vi "datatakersync_master.vi"() -> ()   [LabVIEW 2014, in "filenames.lvlib"]
doc: "This example demonstrates how to acquire a single buffer of voltage measurements using a DAQmx device.\n\nFor instructions on how to connect your signals to the DAQ device, refer to your device documentation."
uses:
  filenames.lvlib
  <resource>/objmgr/daqmx.rc
  <vilib>/DAQmx/configure/timing.llb/DAQmx Timing (Sample Clock).vi
  <vilib>/Utility/error.llb/DialogType.ctl
  <vilib>/DAQmx/create/channels.llb/DAQmx Create Channel (AI-Voltage-Basic).vi
  <vilib>/DAQmx/configure/trigger.llb/DAQmx Start Trigger (Digital Edge).vi
  <vilib>/ptbypt/NI_PtbyPt.lvlib
  <userlib>/Agilis Labview 7.1/AGILIS.llb/enter / leave remote mode.vi
  <vilib>/DAQmx/create/channels.llb/DAQmx Create Channel (AO-Voltage-Basic).vi
  <vilib>/DAQmx/write.llb/DAQmx Write (Analog 1D DBL 1Chan NSamp).vi
  <vilib>/LabVIEW Hacker/LINX/Public/Peripherals/Analog/Analog Read 1 Chan.vi
  <vilib>/Analysis/3filter.llb/Filter Passband Type.ctl
  <vilib>/Analysis/NI_AALBase.lvlib
panel:
  in  "Agilent is negative?":bool
  in  "Set Agilent DC":bool
  in  "stop (DC)":ext=1.0
  in  "start (DC)":ext=1.0
  in  "Number of DC steps":i32=1
  in  "Jog during auto":bool=TRUE
  in  "Move Slide Back 3":bool
  in  "Move Slide  2":bool
  in  "Slide Jog Speed 2":i32(slide) scale=1.0..3.0
  in  "Stop Button":bool=TRUE
  in  "Use interferometer":bool
  out "Motion Direction Indicator":bool
  out "Move Indicator":bool
  in  "Auto Move":bool=TRUE
  in  "Auto Motion Direction":bool
  in  "Tab Control":T1(tab)=enum."I/O"
  out "Indicator Pos 2":bool
  out "Indicator Pos 1":bool=TRUE
  in  "Go to 2":bool
  in  "Go to 1":bool
  in  "Cycles Between Movements":i32=1
  in  "Position 2":dbl=2.5
  in  "Position 1":dbl=-2.5
  out "Main Sig":dbl[][](graph)=[[-1.679588746006175], [-2.01550649520741]]
  out "Main Output":dbl(graph)=1.3000000000000012
  out "Displacement":dbl=1.3000000000000012 format="%#.3f"
  in  "Zero":bool
  in  "Go to Zero":bool
  in  "Automatic":bool
  in  "Motion Direction":bool=TRUE
  in  "Manual Move":bool
  in  "Stop Movement":bool
  in  "Arduino Serial Port":refnum<visa-resource-name>="COM3"
  out "Device Name":string="Arduino Mega 2560"
  in  "Analog Channel":u8
  out "Filtered Signal":dbl(graph)=-1.679588746006175
  in  "filter type":T2=enum."Bandpass"
  in  "order":i32=2
  in  "initialize":bool
  in  "low cutoff freq: fl":dbl=0.45 format="%#_13g"
  out "Raw Signal":dbl(graph)=2.294921875
  in  "Positive Move Steps":i32=30
  in  "Controller Serial Port":u8=6
  in  "Negative Move Steps":i32=30
  in  "Move Period (ms)":u32=10
  in  "high cutoff freq: fh":dbl=1.0
  out "Input Signals":dbl[][](graph)=[[-1.679588746006175], [-2.01550649520741]]
  out "Stepped Signal":dbl(graph)=2.0
  in  "Fringe Counter Settings":T3={"Wavelength"=3.25e-07, "Divisions"=2.0, "Scaling Amplitude"=1.2, "Scaling Offset"=0.0} {"Scaling Offset" format="%0.2f"; "Scaling Amplitude" format="%0.2f"}
  out "Fringe Counter Output Signal":dbl[](graph)=[1.21875e-06]
  out "Relative Displacement":dbl=1.21875e-06
  out "Total Displacement":dbl(graph)=1.3000000000000012
  out "Reset Fringe Counter":bool
  out "Timeout":bool
  in  "Slide Jog Speed":i32(slide) scale=1.0..3.0
  in  "Move Slide":bool
  in  "Move Slide Back":bool
  in  "Error In":errorcluster
  in  "Turn off drive\nwhen flashing?":bool
  in  "set synth":bool
  in  "Sweep type":u16(ring)=1 items=["Chirp", "Single freq", "Both"]
  in  "VISA session":refnum<visa-resource-name>="GPIB0::10::INSTR"
  in  "Physical Channel synth_trigger":tag="Dev5/ao0"
  in  "Digitize on\nother comp?":bool
  in  "stop (F)":ext=100.0
  in  "start (F)":ext=100.0
  in  "Number of F Steps":i32=1
  in  "dc offset?":bool
  in  "volt_div":dbl=200.0
  in  "stop (V)":ext=0.05
  in  "start (V)":ext=0.05
  in  "Number of V Steps":i32=1
  out "error out":errorcluster
  in  "Physical Channel (drive signals)":tag="Dev5/ai0"
  out "Curr threshold":dbl
  in  "Stop threshold":dbl=0.05
  in  "Stop flashing below thresh":bool
  out "Pirani pressure (mbar)":string
  out "CC read error":errorcluster={"status"=FALSE, "code"=1073676294, "source"="VISA Read in read_pressure(SubVI).vi->hdf5(SubVI).vi->filenames.lvlib:datatakersync_master.vi"}
  out "CC pressure (mbar)":string
  out "Pirani read error":errorcluster={"status"=FALSE, "code"=1073676294, "source"="VISA Read in read_pressure(SubVI).vi->hdf5(SubVI).vi->filenames.lvlib:datatakersync_master.vi"}
  in  "# Pulses":i32=3
  in  "Output channel (for flashing)":tag="Dev4/ao0"
  in  "Number of cyles\nbetween flashes":i32=3
  in  "Flash lamp?":bool
  in  "File base name":string="2mbar_zcool"
  in  "Delay time between files(s)":dbl caption="Delay Time (s)"
  in  "Num files":i32=1
  out "Temps (C):":dbl[](array[numeric])
  in  "VISA Refnum in":refnum<visa-resource-name>="GPIB0::19::INSTR"
  in  "Directory path":path=path "D:/Data/20150528/Bead1"
  out "Waveform Graph":dbl[][](graph)
  in  "Number of Samples":i32=100000
  in  "Sample Rate":dbl=10000.0
  in  "Sample Clock Source":tag="/Dev2/PXI_Clk10"
  in  "Terminal Configuration":i32(ring)=-1 items=["default"=-1, "RSE"=10083, "NRSE"=10078, "Differential"=10106, "Pseudodifferential"=12529]
  in  "Max Voltage":dbl=10.0
  in  "Physical Channels (Position signals)":tag="Dev2/ai0:7"
  out "Actual Sample Rate":dbl=10000.0 format="%0.2f"
  # "Channel Settings"
  # "Acquired Data"
  # "Timing Settings"
  # "Flash Lamp Settings"
  # "Pressures and Temperatures"
  # "Logging Settings"
  # "."
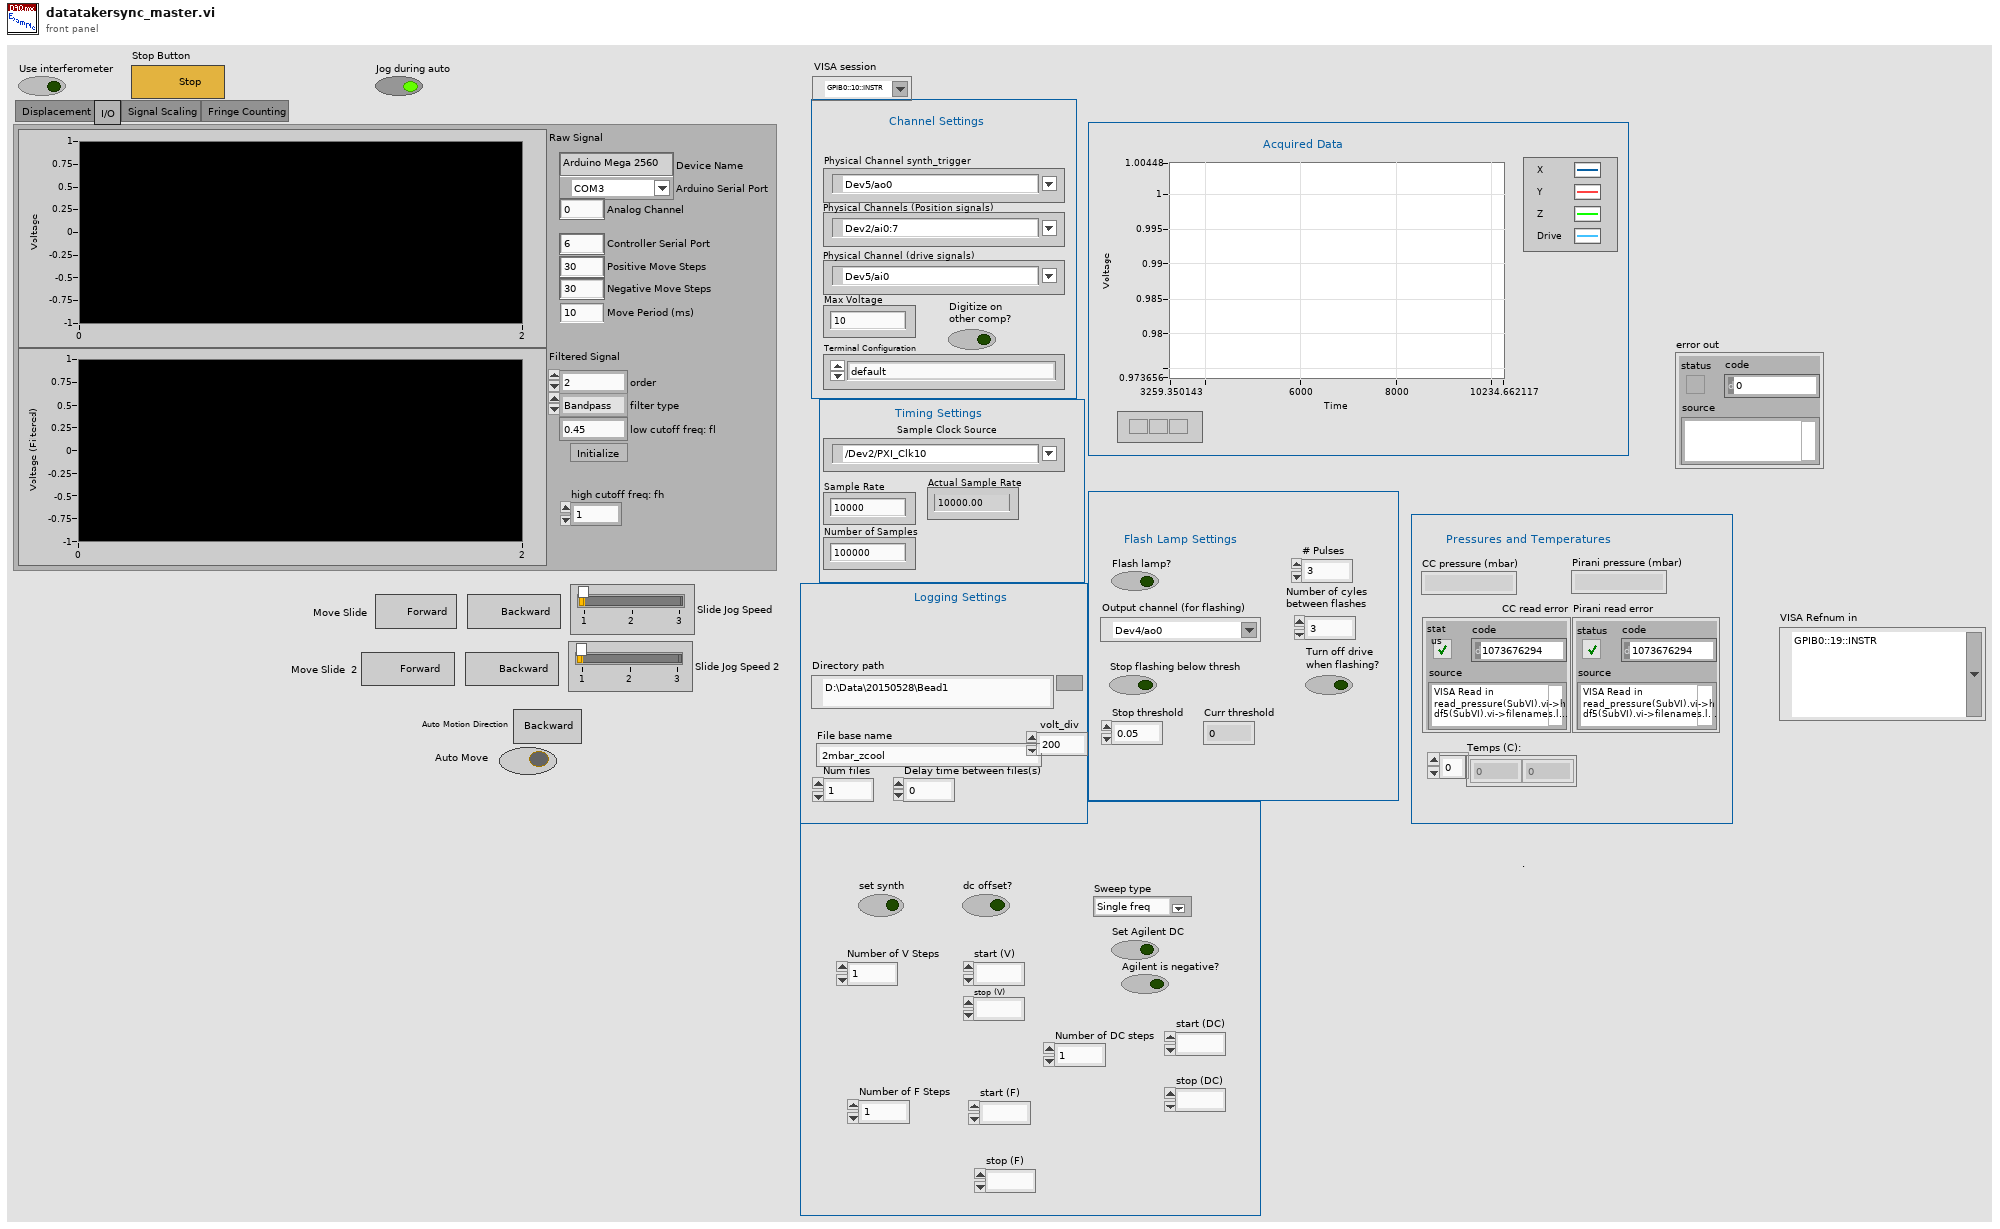
[diagram p1: front panel]
types:
  T1 = enum32{"Displacement", "I/O", "Signal Scaling", "Fringe Counting"}
  T2 = typedef "NI_AALBase.lvlib/Filter Passband Type.ctl" = enum32{"Lowpass", "Highpass", "Bandpass", "Bandstop"}
  T3 = cluster{"Wavelength":dbl, "Divisions":dbl, "Scaling Amplitude":dbl, "Scaling Offset":dbl}
  T4 = typedef "DialogType.ctl" = u16
  T5 = typedef "LVH-LINX.lvlib/LINX Ref.ctl" = cluster{"Platform":T6, "Interface":T7, "LINX Device Config":T8}
  T6 = typedef "LVH-LINX.lvlib/Platform.ctl" = enum16{"LINX", "myRIO"}
  T7 = typedef "LVH-LINX.lvlib/Interface.ctl" = enum16{"Serial", "TCP"}
  T8 = typedef "LVH-LINX.lvlib/Device.lvlib/LINX Device Config.ctl" = cluster{"Interface":T7, "COM Port":refnum<visa-resource-name>, "TCP Configuration":T9, "Device Family":T10, "Device ID":u8, "Device Name":string, "TCP Ref":refnum<k5>}
  T9 = typedef "LVH-LINX.lvlib/Device.lvlib/TCP Config.ctl" = cluster{"IP Address":string, "Port":u16}
  T10 = typedef "LVH-LINX.lvlib/Device Family.ctl" = enum8{"National Instruments", "Digilent", "Arduino"}
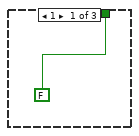
[diagram p3: hidden frame]
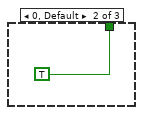
[diagram p4: hidden frame]
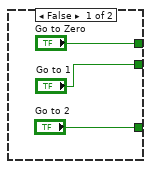
[diagram p5: hidden frame]
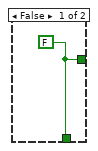
[diagram p6: hidden frame]
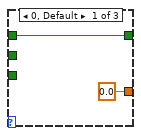
[diagram p8: hidden frame]
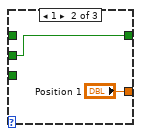
[diagram p9: hidden frame]
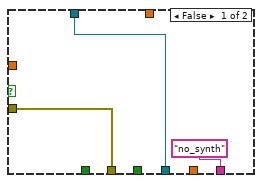
[diagram p11: hidden frame]
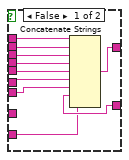
[diagram p12: hidden frame]
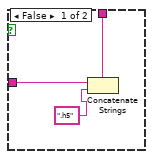
[diagram p14: hidden frame]
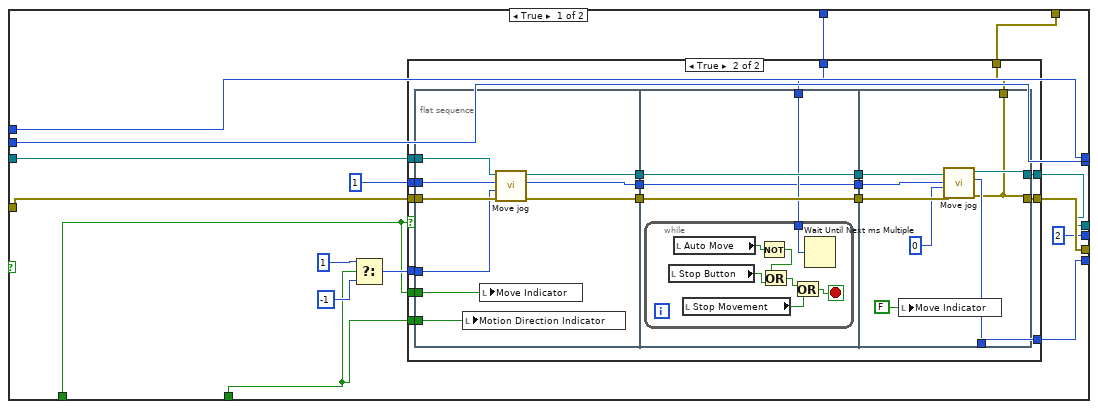
[diagram p18: hidden frame]
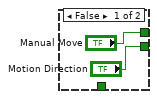
[diagram p20: hidden frame]
diagram:
  w17 = TRUE  # ID Query
  w52 = 10178 items=["Finite Samples"=10178, "Continuous Samples"=10123, "Hardware Timed Single Point"=12522]  # Sample Mode
  n1 = case shown="True" "set synth" {
    tunnel: w17 -> [_ w60]
    tunnel: [refnum<visa-resource-name> refnum ("dup VISA session") w57] -> w16
    tunnel: [errorcluster {"status"=FALSE, "code"=0, "source"=""} ("error out") w56] -> w15
    frame False {
    }
    frame True {
      n2 = call "ag33xxx - Initialize.vi"("ID Query (T: Check)"=w60, "Instrument Resource Name"="VISA session") -> ("error out"=w59:errorcluster, "dup VISA session"=w58:refnum<visa-resource-name>)  [unwired: 8 in]
      n3 = VISA Write(VISA resource name=w58, write buffer="SOUR:BM:NCYC INF;:SOUR:BM:PHAS 0;SOUR INT;:TRIG:SOUR EXT;:SOUR:BM:INT:RATE 1.000000;:BM:STAT ON;", error in (no error)=w59) -> (VISA resource name out=w57:refnum<visa-resource-name>, error out=w56:errorcluster)  [unwired: 1 out]
    }
  }
  n4 = call <vilib>:"Check if File or Folder Exists.vi"("path"="Directory path") -> ("file or folder exists?"=w42:bool, "dup path"=w41:path)  [unwired: 8 in, 1 out]
  n5 = Subtract(x="stop (DC)", y="start (DC)") -> (x-y=w5:ext)
  n6 = case shown="False" w42 {
    tunnel: w41 -> [w63 w68]
    tunnel: [w62 w68] -> w40
    frame False {
      n7 = flat-sequence {
        tunnel: w63 -> [w67]
        tunnel: [w66] -> w62
        frame #0 {
          n8 = call "Create folder?"() -> ("OK"=w65:bool)  [unwired: 18 in, 1 out]
          n9 = Not(x=w65) -> (.not. x?=w64:bool)
          n10 = Stop(stop? (T)=w64) -> ()
        }
        frame #1 {
          n11 = Create Folder(path (use dialog)=w67) -> (created path=w66:path)  [unwired: 2 in, 2 out]
        }
      }
    }
    frame True {
    }
  }
  n12 = Subtract(x="stop (F)", y="start (F)") -> (x-y=w28:ext)
  n13 = Divide(x=w5, y="Number of DC steps") -> (x/y=w4:ext)
  n14 = Divide(x=w28, y="Number of F Steps") -> (x/y=w27:ext)
  n15 = Subtract(x="stop (V)", y="start (V)") -> (x-y=w35:ext)
  n16 = Multiply(x="Max Voltage", y=-1.0) -> (x*y=w45:dbl)
  n17 = Divide(x=w35, y="Number of V Steps") -> (x/y=w33:ext)
  n18 = case shown="True" "Digitize on\nother comp?" {
    selector: "Digitize on\nother comp?" -> [w69 w72]
    tunnel: [errorcluster {"status"=FALSE, "code"=0, "source"=""} ("error out") w75] -> w24
    tunnel: [refnum<k5> refnum ("connection ID") w74] -> w23
    tunnel: [w69 w72] -> w19
    frame False {
    }
    frame True {
      w76 = 60000  # timeout ms
      n19 = call <vilib>:"TCP Listen.vi"("timeout ms (wait forever: -1)"=w76, "port"=u16 6340) -> ("error out"=w75:errorcluster, "connection ID"=w74:refnum<k5>)  [unwired: 5 in, 3 out]
    }
  }
  n20 = local write "Automatic"(FALSE ("Go to Zero")) -> ()
  n21 = for {
    N: "Number of DC steps" -> [_]
    tunnel: w52 -> [w116]
    tunnel: "Physical Channels (Position signals)" -> [w115]
    tunnel: "Terminal Configuration" -> [w114]
    tunnel: "Sample Clock Source" -> [w113]
    tunnel: "Sample Rate" -> [w112]
    tunnel: "Number of Samples" -> [w111]
    tunnel: w45 -> [w110]
    tunnel: "Max Voltage" -> [w109]
    tunnel: w40 -> [w108]
    tunnel: "File base name" -> [w107]
    tunnel: "Output channel (for flashing)" -> [w106]
    tunnel: "Physical Channel (drive signals)" -> [w105]
    tunnel: "Number of V Steps" -> [w104]
    tunnel: w33 -> [w103]
    tunnel: "start (V)" -> [w102]
    tunnel: "Num files" -> [w101]
    tunnel: "volt_div" -> [w100]
    tunnel: w27 -> [w99]
    tunnel: "start (F)" -> [w98]
    tunnel: "Number of F Steps" -> [w97]
    tunnel: w24 -> [w96]
    tunnel: w23 -> [w95]
    tunnel: [w94] -> w22
    tunnel: [w93] -> w21
    tunnel: w19 -> [w92]
    tunnel: [w91] -> w7
    tunnel: "Physical Channel synth_trigger" -> [w90]
    tunnel: w16 -> [w89]
    tunnel: w15 -> [w88]
    tunnel: [w87] -> w14
    tunnel: [w86] -> w13
    tunnel: [w85] -> w12
    tunnel: "Sweep type" -> [w84]
    tunnel: "set synth" -> [w83]
    tunnel: "start (DC)" -> [w81]
    tunnel: w4 -> [w79]
    tunnel: [w77] -> w1
    i -> [w82]
    n22 = Multiply(x=w79, y=w82) -> (x*y=w80:ext)
    n23 = Add(x=w81, y=w80) -> (x+y=w78:ext)
    n24 = for {
      N: w101 -> [_]
      tunnel: w116 -> [w156]
      tunnel: w115 -> [w155]
      tunnel: w114 -> [w154]
      tunnel: w113 -> [w153]
      tunnel: w112 -> [w152]
      tunnel: w111 -> [w151]
      tunnel: w110 -> [w150]
      tunnel: w109 -> [w149]
      tunnel: w108 -> [w148]
      tunnel: w107 -> [w147]
      tunnel: w106 -> [w146]
      tunnel: w105 -> [w145]
      tunnel: w104 -> [w144]
      tunnel: w103 -> [w143]
      tunnel: w102 -> [w142]
      tunnel: w101 -> [w141]
      tunnel: w83 -> [w140]
      tunnel: w100 -> [w139]
      tunnel: w99 -> [w138]
      tunnel: w98 -> [w137]
      tunnel: w97 -> [w136]
      tunnel: w96 -> [w135]
      tunnel: w95 -> [w134]
      tunnel: [w133] -> w94
      tunnel: [w132] -> w93
      tunnel: w92 -> [w131]
      tunnel: [w130] -> w91
      tunnel: w90 -> [w129]
      tunnel: w89 -> [w128]
      tunnel: w88 -> [w127]
      tunnel: [w126] -> w87
      tunnel: [w125] -> w86
      tunnel: [w124] -> w85
      tunnel: w83 -> [w123]
      tunnel: w84 -> [w121]
      tunnel: w78 -> [w119]
      tunnel: [w117] -> w77
      i -> [w120]
      n25 = case shown="2" w121 {
        tunnel: [FALSE TRUE w159] -> w122
        tunnel: w120 -> [_ _ w163]
        frame 1 {
        }
        frame 0, Default {
        }
        frame 2 {
          n26 = Quotient & Remainder(x=w163, y=2) -> (x-y*floor(x/y)=w161:i32)  [unwired: 1 out]
          n27 = Equal?(x=w161, y=0) -> (x = y?=w159:bool)
        }
      }
      n28 = for {
        N: w144 -> [_]
        tunnel: w156 -> [w203]
        tunnel: w155 -> [w202]
        tunnel: w154 -> [w201]
        tunnel: w153 -> [w200]
        tunnel: w152 -> [w199]
        tunnel: w151 -> [w198]
        tunnel: w150 -> [w197]
        tunnel: w149 -> [w196]
        tunnel: w148 -> [w195]
        tunnel: w147 -> [w194]
        tunnel: w146 -> [w193]
        tunnel: w145 -> [w192]
        tunnel: w143 -> [w191]
        tunnel: w142 -> [w190]
        tunnel: w120 -> [w188]
        tunnel: w141 -> [w187]
        tunnel: w140 -> [w186]
        tunnel: w139 -> [w185]
        tunnel: w138 -> [w184]
        tunnel: w137 -> [w183]
        tunnel: w136 -> [w182]
        tunnel: w122 -> [w181]
        tunnel: w135 -> [w180]
        tunnel: w134 -> [w179]
        tunnel: [w178] -> w133
        tunnel: [w177] -> w132
        tunnel: w131 -> [w176]
        tunnel: [w175] -> w130
        tunnel: w129 -> [w174]
        tunnel: w128 -> [w173]
        tunnel: w127 -> [w172]
        tunnel: [w171] -> w126
        tunnel: [w170] -> w125
        tunnel: [w169] -> w124
        tunnel: w123 -> [w168]
        tunnel: w120 -> [w167]
        tunnel: w119 -> [w166]
        tunnel: "Set Agilent DC" -> [w165]
        tunnel: [w164] -> w117
        i -> [w189]
        n29 = for {
          N: w182 -> [_]
          tunnel: w203 -> [w344]
          tunnel: w202 -> [w343]
          tunnel: w201 -> [w342]
          tunnel: w200 -> [w341]
          tunnel: w199 -> [w269]
          tunnel: w198 -> [w340]
          tunnel: w197 -> [w339]
          tunnel: w196 -> [w338]
          tunnel: w195 -> [w337]
          tunnel: w194 -> [w336]
          tunnel: w193 -> [w335]
          tunnel: w192 -> [w334]
          tunnel: w191 -> [w333]
          tunnel: w190 -> [w331]
          tunnel: w189 -> [w329]
          tunnel: w188 -> [w328]
          tunnel: w187 -> [w297]
          tunnel: w186 -> [w327]
          tunnel: w185 -> [w326]
          tunnel: w184 -> [w322]
          tunnel: w183 -> [w321]
          tunnel: w181 -> [w319]
          tunnel: w180 -> [w318]
          tunnel: w179 -> [w317]
          tunnel: [w316] -> w178
          tunnel: [w315] -> w177
          tunnel: w176 -> [w314]
          tunnel: [w313] -> w175
          tunnel: w174 -> [w268]
          tunnel: w173 -> [w264]
          tunnel: w172 -> [w263]
          tunnel: [w259] -> w171
          tunnel: [w255] -> w170
          tunnel: [w254] -> w169
          tunnel: w168 -> [w250]
          tunnel: w167 -> [w212]
          tunnel: w166 -> [w211]
          tunnel: w165 -> [w208]
          tunnel: [w204] -> w164
          i -> [w320]
          n30 = Multiply(x=w322, y=w320) -> (x*y=w323:ext)
          n31 = Add(x=w321, y=w323) -> (x+y=w324:ext)
          n32 = Multiply(x=w329, y=w333) -> (x*y=w332:ext)
          n33 = Add(x=w331, y=w332) -> (x+y=w330:ext)
          n34 = flat-sequence {
            tunnel: w250 -> [w353]
            tunnel: w263 -> [w354]
            tunnel: w264 -> [w355]
            tunnel: w268 -> [w356]
            tunnel: w314 -> [w357]
            tunnel: w317 -> [w358]
            tunnel: w318 -> [w359]
            tunnel: w319 -> [w360]
            tunnel: "dc offset?" -> [w361]
            tunnel: w327 -> [w362]
            tunnel: w328 -> [w363]
            tunnel: w330 -> [w364]
            tunnel: w330 -> [w365]
            tunnel: w324 -> [w366]
            tunnel: w334 -> [w367]
            tunnel: w335 -> [w368]
            tunnel: w336 -> [w369]
            tunnel: w337 -> [w370]
            tunnel: w338 -> [w371]
            tunnel: w339 -> [w372]
            tunnel: w341 -> [w373]
            tunnel: w342 -> [w374]
            tunnel: w343 -> [w375]
            tunnel: [w375] -> w235
            tunnel: [w374] -> w234
            tunnel: [w373] -> w233
            tunnel: [w372] -> w232
            tunnel: [w371] -> w231
            tunnel: [w370] -> w230
            tunnel: [w369] -> w229
            tunnel: [w368] -> w228
            tunnel: [w367] -> w227
            tunnel: [w366] -> w226
            tunnel: [w365] -> w225
            tunnel: [w364] -> w224
            tunnel: [w363] -> w223
            tunnel: [w362] -> w222
            tunnel: [w361] -> w221
            tunnel: [w360] -> w220
            tunnel: [w359] -> w219
            tunnel: [w358] -> w218
            tunnel: [w357] -> w217
            tunnel: [w356] -> w216
            tunnel: [w355] -> w215
            tunnel: [w354] -> w214
            tunnel: [w353] -> w213
            tunnel: w212 -> [w346]
            tunnel: w211 -> [w345]
            tunnel: [w345] -> w210
            tunnel: [w454] -> w301
            tunnel: [w453] -> w302
            tunnel: [w452] -> w303
            tunnel: [w451] -> w304
            tunnel: [w450] -> w305
            tunnel: [w449] -> w306
            tunnel: [w448] -> w307
            tunnel: [w447] -> w308
            tunnel: [w446] -> w309
            tunnel: [w444] -> w310
            tunnel: [w443] -> w311
            tunnel: [w442] -> w312
            tunnel: [w440] -> w300
            tunnel: [w439] -> w299
            tunnel: [w438] -> w298
            tunnel: [w437] -> w267
            tunnel: [w434] -> w262
            tunnel: [w433] -> w258
            tunnel: [w432] -> w251
            tunnel: [w431] -> w246
            tunnel: [w430] -> w245
            tunnel: [w429] -> w240
            tunnel: w235 -> [w454]
            tunnel: w234 -> [w453]
            tunnel: w233 -> [w452]
            tunnel: w232 -> [w451]
            tunnel: w231 -> [w450]
            tunnel: w230 -> [w449]
            tunnel: w229 -> [w448]
            tunnel: w228 -> [w447]
            tunnel: w227 -> [w446]
            tunnel: w226 -> [w444]
            tunnel: w225 -> [w445]
            tunnel: w224 -> [w443]
            tunnel: w223 -> [w442]
            tunnel: w222 -> [w441]
            tunnel: w221 -> [w429]
            tunnel: w220 -> [w431]
            tunnel: w219 -> [w440]
            tunnel: w218 -> [w439]
            tunnel: w217 -> [w438]
            tunnel: w216 -> [w437]
            tunnel: w215 -> [w436]
            tunnel: w214 -> [w435]
            tunnel: w213 -> [w432]
            tunnel: w210 -> [w428]
            tunnel: [w428] -> w209
            tunnel: w208 -> [w427]
            tunnel: [w427] -> w207
            tunnel: w312 -> [w523]
            tunnel: w311 -> [w493]
            tunnel: w310 -> [w528]
            tunnel: [w528] -> w296
            tunnel: w309 -> [w537]
            tunnel: [w537] -> w294
            tunnel: w308 -> [w536]
            tunnel: [w536] -> w292
            tunnel: w307 -> [w502]
            tunnel: w306 -> [w504]
            tunnel: w305 -> [w535]
            tunnel: [w535] -> w289
            tunnel: w304 -> [w534]
            tunnel: [w534] -> w287
            tunnel: w303 -> [w533]
            tunnel: [w533] -> w285
            tunnel: w302 -> [w532]
            tunnel: [w532] -> w283
            tunnel: w301 -> [w531]
            tunnel: [w531] -> w281
            tunnel: w300 -> [w513]
            tunnel: [w510] -> w279
            tunnel: w299 -> [w514]
            tunnel: [w511] -> w277
            tunnel: w298 -> [w512]
            tunnel: [w509] -> w275
            tunnel: [w529] -> w273
            tunnel: w297 -> [w526]
            tunnel: [w523] -> w271
            tunnel: w267 -> [w508]
            tunnel: [w508] -> w265
            tunnel: w262 -> [w507]
            tunnel: [w507] -> w260
            tunnel: w258 -> [w506]
            tunnel: [w506] -> w256
            tunnel: [w505] -> w253
            tunnel: w251 -> [w505]
            tunnel: [w504] -> w249
            tunnel: [w503] -> w248
            tunnel: w246 -> [w496]
            tunnel: w245 -> [w495]
            tunnel: [w496] -> w243
            tunnel: [w495] -> w242
            tunnel: w240 -> [w494]
            tunnel: [w494] -> w239
            tunnel: [w493] -> w237
            tunnel: w209 -> [w491]
            tunnel: w207 -> [w487]
            tunnel: [w487] -> w205
            tunnel: w296 -> [w602]
            tunnel: [w602] -> w295
            tunnel: w294 -> [w601]
            tunnel: [w601] -> w293
            tunnel: w292 -> [w600]
            tunnel: [w600] -> w291
            tunnel: [w599] -> w290
            tunnel: w289 -> [w598]
            tunnel: [w598] -> w288
            tunnel: w287 -> [w597]
            tunnel: [w597] -> w286
            tunnel: w285 -> [w596]
            tunnel: [w596] -> w284
            tunnel: w283 -> [w595]
            tunnel: [w595] -> w282
            tunnel: w281 -> [w589]
            tunnel: [w589] -> w280
            tunnel: w279 -> [w594]
            tunnel: [w594] -> w278
            tunnel: w277 -> [w593]
            tunnel: [w593] -> w276
            tunnel: w275 -> [w592]
            tunnel: [w592] -> w274
            tunnel: w273 -> [w591]
            tunnel: [w591] -> w272
            tunnel: w271 -> [w590]
            tunnel: [w590] -> w270
            tunnel: [w588] -> w266
            tunnel: w265 -> [w588]
            tunnel: [w587] -> w261
            tunnel: w260 -> [w587]
            tunnel: [w586] -> w257
            tunnel: w256 -> [w586]
            tunnel: w253 -> [w585]
            tunnel: [w585] -> w252
            tunnel: w249 -> [w599]
            tunnel: w248 -> [w584]
            tunnel: [w584] -> w247
            tunnel: [w583] -> w244
            tunnel: w243 -> [w583]
            tunnel: w242 -> [w582]
            tunnel: [w582] -> w241
            tunnel: w239 -> [w581]
            tunnel: [w581] -> w238
            tunnel: w237 -> [w580]
            tunnel: [w580] -> w236
            tunnel: [w579] -> w206
            tunnel: w205 -> [w579]
            tunnel: w344 -> [w706]
            tunnel: w269 -> [w626]
            tunnel: w340 -> [w703]
            tunnel: w326 -> [w656]
            tunnel: w295 -> [w616]
            tunnel: w293 -> [w699]
            tunnel: w291 -> [w700]
            tunnel: w290 -> [w650]
            tunnel: w288 -> [w701]
            tunnel: w286 -> [w702]
            tunnel: w284 -> [w648]
            tunnel: w282 -> [w704]
            tunnel: w280 -> [w705]
            tunnel: w278 -> [w652]
            tunnel: w276 -> [w653]
            tunnel: [w652] -> w316
            tunnel: [w653] -> w315
            tunnel: w274 -> [w651]
            tunnel: [w651] -> w313
            tunnel: w272 -> [w655]
            tunnel: w270 -> [w654]
            tunnel: w266 -> [w649]
            tunnel: w261 -> [w611]
            tunnel: [w610] -> w259
            tunnel: w257 -> [w615]
            tunnel: [w609] -> w255
            tunnel: [w634] -> w254
            tunnel: w252 -> [w634]
            tunnel: w247 -> [w633]
            tunnel: w244 -> [w614]
            tunnel: w241 -> [w613]
            tunnel: w238 -> [w612]
            tunnel: w236 -> [w608]
            tunnel: w206 -> [w603]
            tunnel: [w603] -> w204
            frame #0 {
              n35 = case shown="True" "Automatic" {
                tunnel: w346 -> [_ w386]
                tunnel: ["Go to Zero" FALSE ("Go to Zero")] -> w349
                tunnel: ["Go to 1" w380] -> w350
                tunnel: ["Go to 2" w381] -> w351
                frame False {
                }
                frame True {
                  n36 = Quotient & Remainder(x=w386, y="Cycles Between Movements") -> (x-y*floor(x/y)=w384:i32, floor(x/y)=w382:i32)
                  n37 = Equal To 0?(x=w384) -> (x = 0?=w383:bool)
                  n38 = case shown="True" w383 {
                    tunnel: w382 -> [_ w392]
                    tunnel: [w387 w389] -> w381
                    tunnel: [w387 w388] -> w380
                    frame False {
                      w387 = FALSE
                    }
                    frame True {
                      n39 = Quotient & Remainder(x=w392, y=2) -> (x-y*floor(x/y)=w390:i32)  [unwired: 1 out]
                      n40 = Equal To 0?(x=w390) -> (x = 0?=w388:bool)
                      n41 = Not(x=w388) -> (.not. x?=w389:bool)
                    }
                  }
                }
              }
              n42 = local read "Displacement"() -> (w348:dbl)
              n43 = for {
                N: 3 -> [_]
                tunnel: w349 -> [w398]
                tunnel: w350 -> [w395]
                tunnel: w351 -> [w394]
                tunnel: w348 -> [w396]
                i -> [w399]
                n44 = case shown="2" w399 {
                  tunnel: w398 -> [w422 _ _]
                  tunnel: w395 -> [_ w424 _]
                  tunnel: w394 -> [_ _ w426]
                  tunnel: [w422 w424 w426] -> w393
                  tunnel: [0.0 ("Position 2") "Position 1" "Position 2"] -> w397
                  frame 0, Default {
                  }
                  frame 1 {
                  }
                  frame 2 {
                  }
                }
                n45 = case shown="True" w393 {
                  tunnel: w397 -> [_ w406]
                  tunnel: w396 -> [_ w405]
                  tunnel: w395 -> [_ w401]
                  tunnel: w394 -> [_ w402]
                  tunnel: w393 -> [_ w400]
                  frame False {
                  }
                  frame True {
                    n46 = Greater?(x=w406, y=w405) -> (0:w404:bool)
                    n47 = local write "Auto Motion Direction"(w404) -> ()
                    n48 = local write "Auto Move"(w400) -> ()
                    n49 = while {
                      tunnel: w406 -> [w407]
                      tunnel: w404 -> [w419]
                      tunnel: w402 -> [w416]
                      tunnel: w401 -> [w415]
                      tunnel: [FALSE] -> w403
                      stop <- w412 stop-if-true
                      n50 = local read "Displacement"() -> (w408:dbl)
                      n51 = Not Equal?(x=w408, y=w407) -> (x != y?=w409:bool)
                      n52 = Greater?(x=w407, y=w408) -> (0:w420:bool)
                      n53 = Equal?(x=w420, y=w419) -> (x = y?=w414:bool)
                      n54 = And(x=w409, y=w414) -> (x .and. y?=w410:bool)
                      n55 = And(x=w415, y=w410) -> (x .and. y?=→"Indicator Pos 1":bool)
                      n56 = And(x=w416, y=w410) -> (x .and. y?=→"Indicator Pos 2":bool)
                      n57 = Compound Arithmetic op=OR(invert w410, "Stop Movement") -> (w412:bool)
                    }
                    n58 = local write "Auto Move"(w403) -> ()
                  }
                }
              }
            }
            frame #1 {
              n59 = case shown="True" w441 {
                tunnel: w445 -> [_ w471]
                tunnel: w444 -> [_ w470]
                tunnel: w429 -> [_ w469]
                tunnel: w431 -> [_ w468]
                tunnel: w436 -> [w460 w467]
                tunnel: w435 -> [w461 w466]
                tunnel: [w461 w465] -> w434
                tunnel: [w460 w464] -> w433
                tunnel: ["no_synth" ("User Def. Wfm Name") w463] -> w430
                tunnel: w428 -> [_ w462]
                frame False {
                }
                frame True {
                  n60 = flat-sequence {
                    tunnel: w471 -> [w481]
                    tunnel: w470 -> [w480]
                    tunnel: w469 -> [w479]
                    tunnel: w468 -> [w478]
                    tunnel: w467 -> [w477]
                    tunnel: w466 -> [w473]
                    tunnel: [w472] -> w465
                    tunnel: [w476] -> w464
                    tunnel: [w475] -> w463
                    tunnel: w462 -> [w474]
                    frame #0 {
                      w475 = "RANDFREQ" ("User Def. Wfm Name")
                      n61 = call "synth_set(SubVI).vi"("dc offset?"=w479, "dc offset"=w474, "error in (no error)"=w473, "User Def. Wfm Name"=w475, "chirp?"=w478, "VISA session"=w477, "amplitude (V)"=w481, "frequency (Hz)"=w480) -> ("dup VISA session"=w476:refnum<visa-resource-name>, "error out"=w472:errorcluster)  [unwired: 2 in]
                    }
                    frame #1 {
                      n62 = call "Time Delay2"() -> ()  [unwired: 11 in, 1 out]
                    }
                  }
                }
              }
              n63 = case shown="True" w427 {
                tunnel: w428 -> [_ w458]
                frame False {
                }
                frame True {
                  n64 = call <instrlib>:"Agilent E364X Series Output Single Channel DC Volts.vi"("VISA resource name"=refnum<visa-resource-name> "GPIB0::8::INSTR", "Output Enabled (False)"=TRUE, "Voltage Level (0.0 Volts)"=w458, "Current Limit (0 Amps)"=0.01) -> ()  [unwired: 11 in, 1 out]
                }
              }
            }
            frame #2 {
              n65 = Multiply(x=w493, y=ext 1000.0) -> (x*y=w529:ext)
              n66 = Multiply(x=w491, y=ext 1000.0) -> (x*y=w490:ext)
              n67 = Number To Decimal String(number=w490) -> (decimal integer string=w484:string)  [unwired: 1 in]
              n68 = Number To Decimal String(number=w529) -> (decimal integer string=w500:string)  [unwired: 1 in]
              n69 = Number To Decimal String(number=w528) -> (decimal integer string=w498:string)  [unwired: 1 in]
              n70 = Concatenate Strings("-" ("string"), w484) -> (w483:string)
              n71 = Select(t=w483, s="Agilent is negative?", f=w484) -> (s? t:f=w486:string)
              n72 = case shown="True" w496 {
                tunnel: [w547 w551] -> w524
                tunnel: w502 -> [w546 w556]
                tunnel: "_" ("string") -> [w545 w555]
                tunnel: w500 -> [w544 w554]
                tunnel: "mV_" ("string") -> [w543 w553]
                tunnel: w498 -> [w542 _]
                tunnel: "Hz" ("string") -> [w541 _]
                tunnel: w495 -> [_ w552]
                tunnel: "_" ("string") -> [w540 w550]
                tunnel: w486 -> [_ w549]
                tunnel: "mVDC" ("string") -> [w538 w548]
                tunnel: w486 -> [w539 _]
                frame False {
                  n73 = Concatenate Strings(w546, w545, w544, w543, w542, w541, w540, w539, w538) -> (w547:string)
                }
                frame True {
                  n74 = Concatenate Strings(w556, w555, w554, w553, w552, w550, w549, w548) -> (w551:string)
                }
              }
              n75 = Greater?(x=w526, y=1) -> (0:w525:bool)
              n76 = case shown="True" w525 {
                tunnel: w523 -> [_ w578]
                tunnel: [w572 w577] -> w522
                tunnel: w524 -> [w571 w576]
                frame False {
                  n77 = Concatenate Strings(w571, ".h5" ("string")) -> (w572:string)
                }
                frame True {
                  n78 = Number To Decimal String(number=w578) -> (decimal integer string=w574:string)  [unwired: 1 in]
                  n79 = Concatenate Strings(w576, "_" ("string"), w574, ".h5" ("string")) -> (w577:string)
                }
              }
              n80 = Build Path(base path=w504, name or relative path=w522) -> (appended path=w503:path)
              n81 = Path To String(path=w503) -> (string=w519:string)
              n82 = Search and Replace String(input string=w519, search string=".h5", replace string="_drive.h5" ("substring (\"\")")) -> (result string=w518:string)  [unwired: 5 in, 3 out]
              n83 = Search and Replace String(input string=w518, search string="D:", replace string="C:" ("replace string (\"\")")) -> (result string=w515:string)  [unwired: 5 in, 3 out]
              n84 = case shown="True" w512 {
                selector: w512 -> [w557 w560]
                tunnel: w513 -> [w558 w569]
                tunnel: w514 -> [w559 w568]
                tunnel: w515 -> [_ w567]
                tunnel: [w558 w562] -> w510
                tunnel: [w559 w561] -> w511
                tunnel: [w557 w560] -> w509
                frame False {
                }
                frame True {
                  n85 = String Length(string=w567) -> (length=w564:i32)
                  n86 = Type Cast(x=w564) -> (*(type *) &x=w563:string)  [unwired: 1 in]
                  n87 = TCP Write(connection ID=w568, data in=w563, error in (no error)=w569) -> (connection ID out=w566:refnum<k5>, error out=w565:errorcluster)  [unwired: 1 in, 1 out]
                  n88 = TCP Write(connection ID=w566, data in=w567, error in (no error)=w565) -> (connection ID out=w561:refnum<k5>, error out=w562:errorcluster)  [unwired: 1 in, 1 out]
                }
              }
            }
            frame #3 {
              n89 = call "Time Delay3"() -> ()  [unwired: 11 in, 1 out]
            }
            frame #4 {
              w640 = T4 3 items=["no dialog", "OK message", "continue or stop message", "OK message + warnings", "continue/stop + warnings"] ("type of dialog (OK msg:1)")
              w668 = T4 3 items=["no dialog", "OK message", "continue or stop message", "OK message + warnings", "continue/stop + warnings"] ("type of dialog (OK msg:1)")
              w691 = T4 3 items=["no dialog", "OK message", "continue or stop message", "OK message + warnings", "continue/stop + warnings"] ("type of dialog (OK msg:1)")
              # "Acquire Data"
              # "Acquire Data"
              n90 = flat-sequence {
                tunnel: w626 -> [w732]
                tunnel: w648 -> [w736]
                tunnel: w649 -> [w737]
                tunnel: "# Pulses" -> [w734]
                tunnel: w604 -> [w735]
                tunnel: w699 -> [w738]
                tunnel: w700 -> [w733]
                tunnel: w701 -> [w739]
                tunnel: w702 -> [w740]
                tunnel: w703 -> [w741]
                tunnel: w704 -> [w742]
                tunnel: w705 -> [w743]
                tunnel: [w743] -> w625
                tunnel: [w742] -> w624
                tunnel: [w741] -> w623
                tunnel: [w740] -> w622
                tunnel: [w739] -> w621
                tunnel: [w738] -> w620
                tunnel: [w737] -> w619
                tunnel: [w736] -> w618
                tunnel: [w732] -> w617
                tunnel: w616 -> [w730]
                tunnel: w615 -> [w729]
                tunnel: w614 -> [w728]
                tunnel: w613 -> [w727]
                tunnel: w612 -> [w726]
                tunnel: w611 -> [w725]
                tunnel: [w722] -> w610
                tunnel: [w719] -> w609
                tunnel: w608 -> [w714]
                tunnel: w605 -> [w709]
                tunnel: w706 -> [w839]
                tunnel: [w832] -> w690
                tunnel: [w819] -> w678
                tunnel: [w818] -> w677
                tunnel: [w817] -> w676
                tunnel: [w816] -> w675
                tunnel: [w799] -> w647
                tunnel: [w798] -> w644
                tunnel: w625 -> [w838]
                tunnel: w624 -> [w837]
                tunnel: w623 -> [w836]
                tunnel: w622 -> [w835]
                tunnel: w621 -> [w834]
                tunnel: w620 -> [w833]
                tunnel: w619 -> [w809]
                tunnel: w618 -> [w803]
                tunnel: w617 -> [w797]
                frame #0 {
                  n91 = flat-sequence {
                    tunnel: w734 -> [w753]
                    tunnel: [w753] -> w731
                    tunnel: w730 -> [w747]
                    tunnel: w729 -> [w752]
                    tunnel: w728 -> [w748]
                    tunnel: w727 -> [w746]
                    tunnel: w726 -> [w745]
                    tunnel: w725 -> [w751]
                    tunnel: [w750] -> w723
                    tunnel: [w749] -> w720
                    tunnel: [w748] -> w718
                    tunnel: [w747] -> w716
                    tunnel: [w746] -> w713
                    tunnel: [w745] -> w711
                    tunnel: w709 -> [w744]
                    tunnel: [w744] -> w707
                    tunnel: w735 -> [w775]
                    tunnel: w733 -> [w773]
                    tunnel: w732 -> [w772]
                    tunnel: w731 -> [w774]
                    tunnel: [w771] -> w724
                    tunnel: w723 -> [w771]
                    tunnel: [w770] -> w721
                    tunnel: w720 -> [w770]
                    tunnel: w718 -> [w769]
                    tunnel: [w769] -> w717
                    tunnel: w716 -> [w768]
                    tunnel: [w768] -> w715
                    tunnel: w713 -> [w767]
                    tunnel: [w767] -> w712
                    tunnel: w711 -> [w766]
                    tunnel: [w766] -> w710
                    tunnel: [w765] -> w708
                    tunnel: w707 -> [w765]
                    tunnel: w724 -> [w784]
                    tunnel: [w782] -> w722
                    tunnel: w721 -> [w785]
                    tunnel: [w783] -> w719
                    tunnel: w717 -> [w781]
                    tunnel: w715 -> [w780]
                    tunnel: w714 -> [w779]
                    tunnel: w712 -> [w778]
                    tunnel: w710 -> [w777]
                    tunnel: w708 -> [w776]
                    frame #0 {
                      n92 = case shown="True" w744 {
                        tunnel: w752 -> [w755 w763]
                        tunnel: w751 -> [w754 w762]
                        tunnel: [w754 w761] -> w750
                        tunnel: [w755 w760] -> w749
                        tunnel: w748 -> [_ w759]
                        tunnel: w747 -> [_ w758]
                        tunnel: w746 -> [_ w757]
                        tunnel: w745 -> [_ w756]
                        frame False {
                        }
                        frame True {
                          n93 = call "synth_set(SubVI).vi"("dc offset?"=w756, "error in (no error)"=w762, "User Def. Wfm Name"=w757, "chirp?"=w759, "VISA session"=w763, "amplitude (V)"=ext 0.05, "frequency (Hz)"=w758) -> ("dup VISA session"=w760:refnum<visa-resource-name>, "error out"=w761:errorcluster)  [unwired: 3 in]
                          n94 = call "Time Delay4"() -> ()  [unwired: 11 in, 1 out]
                        }
                      }
                    }
                    frame #1 {
                      n95 = call "flasher(SubVI).vi"("Sample Rate"=w772, "# Pulses"=w774, "Boolean"=w775, "Output channel (for flashing)"=w773) -> ()  [unwired: 8 in]
                    }
                    frame #2 {
                      n96 = case shown="True" w776 {
                        tunnel: w785 -> [w786 w796]
                        tunnel: w784 -> [w787 w795]
                        tunnel: [w786 w794] -> w783
                        tunnel: [w787 w793] -> w782
                        tunnel: w781 -> [_ w792]
                        tunnel: w780 -> [_ w791]
                        tunnel: w779 -> [_ w790]
                        tunnel: w778 -> [_ w789]
                        tunnel: w777 -> [_ w788]
                        frame False {
                        }
                        frame True {
                          n97 = call "synth_set(SubVI).vi"("dc offset?"=w788, "error in (no error)"=w795, "User Def. Wfm Name"=w789, "chirp?"=w792, "VISA session"=w796, "amplitude (V)"=w790, "frequency (Hz)"=w791) -> ("dup VISA session"=w794:refnum<visa-resource-name>, "error out"=w793:errorcluster)  [unwired: 3 in]
                          n98 = call "Time Delay5"() -> ()  [unwired: 11 in, 1 out]
                        }
                      }
                    }
                  }
                }
                frame #1 {
                  w804 = 10000000.0 ("RefClk.Rate")
                  # "Trigger Settings"
                  # "Timing Settings"
                  # "Channel Settings"
                  n99 = call-poly <vilib>:"DAQmx Create Virtual Channel.vi"("maximum value"=w834, "minimum value"=w835, "input terminal configuration"=w837, "physical channels"=w833) -> ("task out"=w829:refnum<k21>)  [unwired: 10 in, 1 out]
                  n100 = call-poly <vilib>:"DAQmx Create Virtual Channel.vi"("maximum value"=w834, "minimum value"=w835, "input terminal configuration"=w837, "physical channels"=w838) -> ("task out"=w831:refnum<k21>, "error out"=w830:errorcluster)  [unwired: 10 in]
                  n101 = call-poly <vilib>:"DAQmx Create Virtual Channel.vi"("physical channels"=w809) -> ("task out"=w808:refnum<k21>, "error out"=w806:errorcluster)  [unwired: 13 in]
                  n102 = call-poly <vilib>:"DAQmx Timing.vi"("task/channels in"=w829, "sample mode"=w839, "samples per channel"=w836, "rate"=w797) -> ("task out"=w826:refnum<k21>, "error out"=w825:errorcluster)  [unwired: 10 in]
                  n103 = call-poly <vilib>:"DAQmx Timing.vi"("task/channels in"=w808, "rate"=w797, "error in"=w806) -> ("task out"=w807:refnum<k21>, "error out"=w805:errorcluster)  [unwired: 11 in]
                  n104 = call-poly <vilib>:"DAQmx Timing.vi"("task/channels in"=w831, "sample mode"=w839, "samples per channel"=w836, "rate"=w797, "error in"=w830) -> ("task out"=w828:refnum<k21>, "error out"=w827:errorcluster)  [unwired: 9 in]
                  n105 = property class="DAQmx Timing"(reference=w826, error in=w825, "More:Reference Clock:Source"=w803, "More:Reference Clock:Rate"=w804) -> (reference out=w821:refnum<k21>, error out=w820:errorcluster)
                  n106 = property class="DAQmx Timing"(reference=w828, error in=w827, "More:Reference Clock:Source"=w803, "More:Reference Clock:Rate"=w804) -> (reference out=w824:refnum<k21>, error out=w823:errorcluster)
                  n107 = property class="DAQmx Timing"(reference=w807, error in=w805, "More:Reference Clock:Source"=w803, "More:Reference Clock:Rate"=w804) -> (reference out=w801:refnum<k21>, error out=w802:errorcluster)
                  n108 = property class="DAQmx Timing"(reference=w824, error in=w823) -> (reference out=w815:refnum<k21>, error out=w813:errorcluster, "SampClk.Rate"=w832:dbl)
                  "Actual Sample Rate" <- w832
                  n109 = property class="DAQmx Export Signal"(reference=w815, error in=w813, "StartTrig.OutputTerm"=tag "/Dev2/PFI1", "StartTrig.OutputTerm"=tag "/Dev2/PFI0" ("10MHzRefClk.OutputTerm")) -> (reference out=w814:refnum<k21>, error out=w812:errorcluster)
                  n110 = call "Get Full Terminal Name.vi"("error in (no error)"=w812, "Local Terminal Name"="ai/StartTrigger", "task/channels in"=w814) -> ("error out"=w818:errorcluster, "Terminal Name with Device Prefix"=w800:tag, "task out"=w819:refnum<k21>)  [unwired: 6 in]
                  n111 = call-poly <vilib>:"DAQmx Trigger.vi"("task/channels in"=w821, "source"=w800, "error in"=w820) -> ("task out"=w817:refnum<k21>, "error out"=w816:errorcluster)  [unwired: 11 in]
                  n112 = call-poly <vilib>:"DAQmx Trigger.vi"("task/channels in"=w801, "source"=w800, "error in"=w802) -> ("task out"=w798:refnum<k21>, "error out"=w799:errorcluster)  [unwired: 11 in]
                }
              }
              n113 = call "threshold_stop(SubVI).vi"("Stop threshold"="Stop threshold", "Stop flashing below thresh"="Stop flashing below thresh", "dup path"=w650) -> ("Curr threshold"=→"Curr threshold":dbl, "Boolean"=w682:bool)  [unwired: 7 in]
              n114 = call "flash_cycle(SubVI).vi"("Boolean in"=w682, "Number of cyles\nbetween flashes"="Number of cyles\nbetween flashes", "Numeric"=w654, "Flash lamp?"="Flash lamp?") -> ("Boolean out"=w604:bool)  [unwired: 7 in]
              n115 = And(x="Turn off drive\nwhen flashing?", y=w604) -> (x .and. y?=w605:bool)
              n116 = Select(t="# Pulses", s=w604, f=0) -> (s? t:f=w679:i32)
              n117 = flat-sequence {
                tunnel: w644 -> [w840]
                tunnel: w647 -> [w841]
                tunnel: w675 -> [w842]
                tunnel: w676 -> [w843]
                tunnel: w677 -> [w844]
                tunnel: w678 -> [w845]
                tunnel: [w845] -> w632
                tunnel: [w844] -> w631
                tunnel: [w843] -> w630
                tunnel: [w842] -> w629
                tunnel: [w841] -> w628
                tunnel: [w840] -> w627
                tunnel: [w861] -> w698
                tunnel: [w860] -> w697
                tunnel: [w859] -> w696
                tunnel: [w858] -> w695
                tunnel: [w857] -> w646
                tunnel: [w856] -> w645
                tunnel: w632 -> [w861]
                tunnel: w631 -> [w860]
                tunnel: w630 -> [w863]
                tunnel: w629 -> [w862]
                tunnel: w628 -> [w850]
                tunnel: w627 -> [w852]
                tunnel: [w870] -> w688
                tunnel: [w868] -> w689
                tunnel: w698 -> [w871]
                tunnel: w697 -> [w869]
                tunnel: [w867] -> w674
                tunnel: w696 -> [w867]
                tunnel: [w866] -> w673
                tunnel: w695 -> [w866]
                tunnel: w646 -> [w865]
                tunnel: [w865] -> w637
                tunnel: w645 -> [w864]
                tunnel: [w864] -> w636
                frame #0 {
                }
                frame #1 {
                  n118 = Initialize Array(0.0 ("element"), 100 ("dimension size")) -> (w848:dbl[])
                  n119 = Replace Array Subset(array=w848, new element=5.0 ("new element/subarray"), index=1) -> (w853:dbl[])
                  n120 = call-poly <vilib>:"DAQmx Write.vi"("task/channels in"=w852, "data"=w853, "error in"=w850) -> ("task out"=w851:refnum<k21>, "error out"=w849:errorcluster)  [unwired: 10 in, 1 out]
                  n121 = call <vilib>:"DAQmx Start Task.vi"("task/channels in"=w863, "error in"=w862) -> ("task out"=w859:refnum<k21>, "error out"=w858:errorcluster)  [unwired: 12 in]
                  n122 = call <vilib>:"DAQmx Start Task.vi"("task/channels in"=w851, "error in"=w849) -> ("task out"=w857:refnum<k21>, "error out"=w856:errorcluster)  [unwired: 12 in]
                }
                frame #2 {
                  n123 = call <vilib>:"DAQmx Start Task.vi"("task/channels in"=w871, "error in"=w869) -> ("task out"=w870:refnum<k21>, "error out"=w868:errorcluster)  [unwired: 12 in]
                }
              }
              n124 = call "hdf5(SubVI).vi"("Refnum in"=w688, "VISA Refnum in"="VISA Refnum in", "appended path"=w633, "Max Voltage"=w701, "error out 3"=w673, "f"=w679, "SampClk.Rate"=w690, "error in (no error)"=w689, "drive_amplitude"=w655, "task in"=w674, "drive_freq"=w616, "volt_div"=w656) -> ("task out 4"=w687:refnum<k21>, "Array"=→"Waveform Graph":dbl[][], "CC read error"=→"CC read error":errorcluster, "Refnum out"=w667:refnum<k21>, 21:"error out"=→"error out":errorcluster, "error out 4"=w686:errorcluster, "error out 2"=w666:errorcluster, "Pirani pressure (mbar)"=→"Pirani pressure (mbar)":string, "CC pressure (mbar)"=→"CC pressure (mbar)":string, "Temps (C):"=→"Temps (C):":dbl[], 27:"error out"=→"Pirani read error":errorcluster)  [unwired: 5 in]
              n125 = call <vilib>:"DAQmx Stop Task.vi"("task/channels in"=w687, "error in"=w686) -> ("task out"=w693:refnum<k21>, "error out"=w692:errorcluster)  [unwired: 12 in]
              n126 = call <vilib>:"DAQmx Stop Task.vi"("task/channels in"=w667, "error in"=w666) -> ("task out"=w670:refnum<k21>, "error out"=w669:errorcluster)  [unwired: 12 in]
              n127 = call <vilib>:"DAQmx Wait Until Done.vi"("task/channels in"=w637, "timeout (sec)"=10.0, "error in"=w636) -> ("task out"=w642:refnum<k21>, "error out"=w638:errorcluster)  [unwired: 11 in]
              n128 = call <vilib>:"DAQmx Clear Task.vi"("task in"=w693, "error in"=w692) -> ("error out"=w694:errorcluster)  [unwired: 13 in]
              n129 = call <vilib>:"DAQmx Clear Task.vi"("task in"=w670, "error in"=w669) -> ("error out"=w671:errorcluster)  [unwired: 13 in]
              n130 = call <vilib>:"DAQmx Stop Task.vi"("task/channels in"=w642, "error in"=w638) -> ("task out"=w643:refnum<k21>, "error out"=w639:errorcluster)  [unwired: 12 in]
              n131 = call <vilib>:"DAQmx Clear Task.vi"("task in"=w643, "error in"=w639) -> ("error out"=w641:errorcluster)  [unwired: 13 in]
              n132 = call <vilib>:"Simple Error Handler.vi"("type of dialog (OK msg:1)"=w691, "error in (no error)"=w694) -> ()  [unwired: 3 in, 5 out]
              n133 = call <vilib>:"Simple Error Handler.vi"("type of dialog (OK msg:1)"=w668, "error in (no error)"=w671) -> ()  [unwired: 3 in, 5 out]
              n134 = call <vilib>:"Simple Error Handler.vi"("type of dialog (OK msg:1)"=w640, "error in (no error)"=w641) -> ()  [unwired: 3 in, 5 out]
              n135 = call "Time Delay"("Delay Time (s)"="Delay time between files(s)") -> ()  [unwired: 10 in, 1 out]
            }
          }
        }
      }
    }
  }
  n136 = case shown="True" "Use interferometer" {
    frame False {
    }
    frame True {
      w876 = FALSE ("Move")
      w882 = 0
      n137 = Bundle(FALSE, 0, "") -> (w888:errorcluster)  [unwired: 1 in]
      n138 = call <userlib>:"port init.vi"("SerialPort (1)"="Controller Serial Port") -> ("Visa Handle"=w884:refnum<visa-resource-name>)  [unwired: 3 in, 1 out]
      n139 = local write "Manual Move"(w876) -> ()
      n140 = call "enter / leave remote mode.vi"("error in"=w888, "enter / disable remote mode (True)"=TRUE, "VISA handle in"=w884) -> ("error out"=w885:errorcluster, "VISA handle out"=w886:refnum<visa-resource-name>, "TimeoutFlag"=w887:bool)  [unwired: 6 in]
      n141 = local write "Auto Move"(w876) -> ()
      n142 = local write "Timeout"(w887) -> ()
      n143 = call <vilib>:"Initialize.vi"("Serial Port"="Arduino Serial Port", "Error In"="Error In") -> ("Error Out"=w896:errorcluster, "Device Name"=→"Device Name":string, "LINX Ref"=w897:T5)  [unwired: 7 in]
      n144 = local write "Stop Button"(FALSE ("Stop Button")) -> ()
      n145 = while {
        tunnel: w886 -> [w929]
        shift-right: [w928] -> _
        shift-left: w882 -> [w930]
        shift-right: [w921] -> w879
        shift-left: w885 -> [w922]
        tunnel: [w924] -> w880
        tunnel: [w925] -> w878
        shift-right: [w927] -> _
        shift-left: w882 -> [w926]
        tunnel: [w923] -> w877
        tunnel: "Jog during auto" -> [w917]
        stop <- w918 stop-if-true
        n146 = case shown="False" w917 {
          tunnel: w930 -> [w939 w1034]
          tunnel: w929 -> [w941 w1032]
          tunnel: [w938 w1030] -> w928
          tunnel: [w939 w1022] -> w927
          tunnel: w926 -> [w938 w1021]
          tunnel: [w940 w1013] -> w925
          tunnel: [2 ("Axis out") w1012] -> w924
          tunnel: [w937 w1006] -> w923
          tunnel: w922 -> [w946 w1004]
          tunnel: [w945 w997] -> w921
          tunnel: [w933 w997] -> w919
          tunnel: "Auto Move" -> [w932 w996]
          tunnel: "Auto Motion Direction" -> [w931 w995]
          tunnel: "Move Period (ms)" -> [w934 _]
          frame True {
            n147 = Select(t=1 ("Jog mode"), s=w931, f=-1 ("Jog mode")) -> (s? t:f=w942:i32)
            n148 = case shown="True" w932 {
              tunnel: w946 -> [w947 w962]
              tunnel: [w947 w961] -> w945
              tunnel: w942 -> [_ w960]
              tunnel: w941 -> [w949 w959]
              tunnel: [w949 w958] -> w940
              tunnel: [w948 w953] -> w937
              tunnel: u32 1 ("Axis in") -> [w948 w957]
              tunnel: w934 -> [_ w956]
              tunnel: [w947 w952] -> w933
              tunnel: w932 -> [_ w951]
              tunnel: w931 -> [_ w950]
              frame False {
              }
              frame True {
                n149 = flat-sequence {
                  tunnel: w962 -> [w975]
                  tunnel: w960 -> [w973]
                  tunnel: w959 -> [w972]
                  tunnel: [w974] -> w966
                  tunnel: [w971] -> w965
                  tunnel: w957 -> [w970]
                  tunnel: [w969] -> w954
                  tunnel: w951 -> [w968]
                  tunnel: w950 -> [w967]
                  tunnel: w966 -> [w979]
                  tunnel: w965 -> [w978]
                  tunnel: [w979] -> w964
                  tunnel: [w978] -> w963
                  tunnel: w956 -> [w977]
                  tunnel: [w976] -> w955
                  tunnel: w954 -> [w976]
                  tunnel: [w990] -> w958
                  tunnel: [w988] -> w961
                  tunnel: w964 -> [w993]
                  tunnel: w963 -> [w994]
                  tunnel: w955 -> [w992]
                  tunnel: [w989] -> w953
                  tunnel: [w988] -> w952
                  frame #0 {
                    n150 = local write "Motion Direction Indicator"(w967) -> ()
                    n151 = local write "Move Indicator"(w968) -> ()
                    n152 = call <userlib>:"Move jog.vi"("error in"=w975, "Jog mode"=w973, "Axis in"=w970, "VISA Handle in"=w972) -> ("error out"=w974:errorcluster, "Axis out"=w969:i32, "VISA Handle out"=w971:refnum<visa-resource-name>)  [unwired: 2 in, 1 out]
                  }
                  frame #1 {
                    n153 = while {
                      tunnel: w977 -> [w986]
                      stop <- w982 stop-if-true
                      n154 = local read "Stop Button"() -> (w985:bool)
                      n155 = local read "Auto Move"() -> (w981:bool)
                      n156 = local read "Stop Movement"() -> (w983:bool)
                      n157 = Not(x=w981) -> (.not. x?=w980:bool)
                      n158 = Or(x=w980, y=w985) -> (x .or. y?=w984:bool)
                      n159 = Or(x=w984, y=w983) -> (x .or. y?=w982:bool)
                      n160 = Wait Until Next ms Multiple(millisecond multiple=w986) -> ()  [unwired: 1 out]
                    }
                  }
                  frame #2 {
                    n161 = local write "Move Indicator"(FALSE ("Move Indicator")) -> ()
                    n162 = call <userlib>:"Move jog.vi"("error in"=w993, "Jog mode"=0, "Axis in"=w992, "VISA Handle in"=w994) -> ("error out"=w988:errorcluster, "Axis out"=w989:i32, "VISA Handle out"=w990:refnum<visa-resource-name>)  [unwired: 2 in, 1 out]
                  }
                }
              }
            }
          }
          frame False {
            n163 = Not Equal?(x="Positive Move Steps", y=w1034) -> (x != y?=w1035:bool)
            n164 = Not Equal?(x="Negative Move Steps", y=w1021) -> (x != y?=w1018:bool)
            n165 = case shown="True" w996 {
              selector: w996 -> [_ w1039]
              tunnel: ["Motion Direction" w1038] -> w1024
              tunnel: ["Manual Move" w1039] -> w1003
              tunnel: w995 -> [_ w1038]
              frame False {
              }
              frame True {
              }
            }
            "Move Indicator" <- w1003
            "Motion Direction Indicator" <- w1024
            n166 = Or(x=w1035, y=w1018) -> (x .or. y?=w1019:bool)
            n167 = case shown="True" w1019 {
              tunnel: w1004 -> [w1124 w1138]
              tunnel: w1032 -> [w1123 w1136]
              tunnel: 1 ("Axis in") -> [w1121 w1129]
              tunnel: "Positive Move Steps" -> [_ w1130]
              tunnel: [w1125 w1130] -> w1031
              tunnel: w1034 -> [w1125 _]
              tunnel: [w1124 w1134] -> w1028
              tunnel: [w1123 w1133] -> w1029
              tunnel: "Negative Move Steps" -> [_ w1127]
              tunnel: [w1122 w1127] -> w1023
              tunnel: w1021 -> [w1122 _]
              tunnel: [w1121 w1126] -> w1017
              frame False {
              }
              frame True {
                n168 = call <userlib>:"set positive step size.vi"("error in"=w1138, "Step size (positive direction)"=w1130, "Axis in"=w1129, "VISA Handle in"=w1136) -> ("error out"=w1135:errorcluster, "Axis out"=w1131:i32, "VISA Handle out"=w1132:refnum<visa-resource-name>, "TimeoutFlag"=w1137:bool)  [unwired: 2 in]
                n169 = local write "Timeout"(w1137) -> ()
                n170 = call <userlib>:"set negative step size.vi"("error in"=w1135, "Step size (negative direction)"=w1127, "Axis in"=w1131, "VISA Handle in"=w1132) -> ("error out"=w1134:errorcluster, "Axis out"=w1126:i32, "VISA Handle out"=w1133:refnum<visa-resource-name>, "TimeoutFlag"=w1128:bool)  [unwired: 2 in]
                n171 = local write "Timeout"(w1128) -> ()
              }
            }
            n172 = Select(t=1 ("Number of steps"), s=w1024, f=-1) -> (s? t:f=w1025:i32)
            n173 = Compound Arithmetic op=AND("Move Slide  2", invert "Move Slide Back 3") -> (w998:bool)
            n174 = Compound Arithmetic op=AND("Move Slide Back 3", invert "Move Slide  2") -> (w999:bool)
            n175 = case shown="False" w1003 {
              tunnel: w1031 -> [w1080 w1116]
              tunnel: [w1080 w1116] -> w1030
              tunnel: w1029 -> [w1076 w1117]
              tunnel: [w1075 w1118] -> w1014
              tunnel: w1028 -> [w1077 w1120]
              tunnel: [w1074 w1119] -> w1015
              tunnel: w1025 -> [_ w1115]
              tunnel: w1023 -> [w1079 w1114]
              tunnel: [w1079 w1114] -> w1022
              tunnel: [w1078 w1112] -> w1012
              tunnel: w1017 -> [w1078 w1111]
              tunnel: "Slide Jog Speed 2" -> [w1072 _]
              tunnel: w999 -> [w1071 _]
              tunnel: w998 -> [w1070 _]
              frame False {
                n176 = case shown="False" w1070 {
                  tunnel: w1077 -> [w1086 w1110]
                  tunnel: [w1085 w1109] -> w1074
                  tunnel: w1076 -> [w1084 w1108]
                  tunnel: [w1083 w1107] -> w1075
                  tunnel: w1072 -> [w1088 w1106]
                  tunnel: w1071 -> [w1087 _]
                  tunnel: [w1081 w1105] -> _
                  tunnel: u32 1 ("Axis in") -> [w1082 w1104]
                  frame False {
                    n177 = case shown="True" w1087 {
                      tunnel: w1088 -> [_ w1103]
                      tunnel: w1086 -> [w1089 w1101]
                      tunnel: [w1090 w1100] -> w1085
                      tunnel: w1084 -> [w1092 w1099]
                      tunnel: [w1091 w1098] -> w1083
                      tunnel: w1082 -> [w1095 w1097]
                      tunnel: [w1093 w1096] -> w1081
                      frame False {
                        n178 = call <userlib>:"Move jog.vi"("error in"=w1089, "Jog mode"=0, "Axis in"=w1095, "VISA Handle in"=w1092) -> ("error out"=w1090:errorcluster, "Axis out"=w1093:i32, "VISA Handle out"=w1091:refnum<visa-resource-name>)  [unwired: 2 in, 1 out]
                      }
                      frame True {
                        n179 = Negate(x=w1103) -> (-x=w1102:i32)
                        n180 = call <userlib>:"Move jog.vi"("error in"=w1101, "Jog mode"=w1102, "Axis in"=w1097, "VISA Handle in"=w1099) -> ("error out"=w1100:errorcluster, "Axis out"=w1096:i32, "VISA Handle out"=w1098:refnum<visa-resource-name>)  [unwired: 2 in, 1 out]
                      }
                    }
                  }
                  frame True {
                    n181 = call <userlib>:"Move jog.vi"("error in"=w1110, "Jog mode"=w1106, "Axis in"=w1104, "VISA Handle in"=w1108) -> ("error out"=w1109:errorcluster, "Axis out"=w1105:i32, "VISA Handle out"=w1107:refnum<visa-resource-name>)  [unwired: 2 in, 1 out]
                  }
                }
              }
              frame True {
                n182 = call <userlib>:"move relative.vi"("error in"=w1120, "Number of steps"=w1115, "Axis in"=w1111, "VISA Handle in"=w1117) -> ("error out"=w1119:errorcluster, "Axis out"=w1112:i32, "VISA Handle out"=w1118:refnum<visa-resource-name>, "TimeoutFlag"=w1113:bool)  [unwired: 2 in]
                n183 = local write "Timeout"(w1113) -> ()
              }
            }
            n184 = Compound Arithmetic op=AND("Move Slide", invert "Move Slide Back") -> (w1010:bool)
            n185 = Compound Arithmetic op=AND("Move Slide Back", invert "Move Slide") -> (w1008:bool)
            n186 = case shown="False" w1010 {
              tunnel: w1015 -> [w1045 w1069]
              tunnel: [w1044 w1068] -> w997
              tunnel: w1014 -> [w1043 w1067]
              tunnel: [w1042 w1066] -> w1013
              tunnel: "Slide Jog Speed" -> [w1047 w1065]
              tunnel: w1008 -> [w1046 _]
              tunnel: [w1040 w1064] -> w1006
              tunnel: u32 2 ("Axis in") -> [w1041 w1063]
              frame False {
                n187 = case shown="False" w1046 {
                  tunnel: w1047 -> [_ w1062]
                  tunnel: w1045 -> [w1048 w1060]
                  tunnel: [w1049 w1059] -> w1044
                  tunnel: w1043 -> [w1051 w1058]
                  tunnel: [w1050 w1057] -> w1042
                  tunnel: w1041 -> [w1054 w1056]
                  tunnel: [w1052 w1055] -> w1040
                  frame False {
                    n188 = call <userlib>:"Move jog.vi"("error in"=w1048, "Jog mode"=0, "Axis in"=w1054, "VISA Handle in"=w1051) -> ("error out"=w1049:errorcluster, "Axis out"=w1052:i32, "VISA Handle out"=w1050:refnum<visa-resource-name>)  [unwired: 2 in, 1 out]
                  }
                  frame True {
                    n189 = Negate(x=w1062) -> (-x=w1061:i32)
                    n190 = call <userlib>:"Move jog.vi"("error in"=w1060, "Jog mode"=w1061, "Axis in"=w1056, "VISA Handle in"=w1058) -> ("error out"=w1059:errorcluster, "Axis out"=w1055:i32, "VISA Handle out"=w1057:refnum<visa-resource-name>)  [unwired: 2 in, 1 out]
                  }
                }
              }
              frame True {
                n191 = call <userlib>:"Move jog.vi"("error in"=w1069, "Jog mode"=w1065, "Axis in"=w1063, "VISA Handle in"=w1067) -> ("error out"=w1068:errorcluster, "Axis out"=w1064:i32, "VISA Handle out"=w1066:refnum<visa-resource-name>)  [unwired: 2 in, 1 out]
              }
            }
          }
        }
        n192 = Wait Until Next ms Multiple(millisecond multiple="Move Period (ms)") -> ()  [unwired: 1 out]
        n193 = Or(x="Stop Button", y=w919) -> (x .or. y?=w918:bool)
      }
      n194 = while {
        tunnel: w897 -> [w1177]
        tunnel: [w1176] -> w873
        tunnel: [w1142] -> w874
        tunnel: w896 -> [w1175]
        shift-right: [w1156] -> _
        shift-left: 0.0 ("Displacement") -> [w1148]
        shift-right: [w1157] -> _
        shift-left: _ -> [w1158]
        shift-right: [w1152] -> _
        shift-left: _ -> [w1150]
        stop <- w1144 stop-if-true
        w1171 = 200.0 ("sampling freq: fs")
        n195 = local read "Motion Direction Indicator"() -> (w1149:bool)
        n196 = call-poly <vilib>:"Analog Read.vi"("Error In"=w1175, "Analog Channel"="Analog Channel", "LINX Resource"=w1177) -> ("Error Out"=w1142:errorcluster, "AI Value"=w1164:dbl, "LINX Resource"=w1176:T5)  [unwired: 5 in, 1 out]
        "Raw Signal" <- w1164
        n197 = local read "Move Indicator"() -> (w1159:bool)
        n198 = Select(t=0.0, s="Zero", f=w1148) -> (s? t:f=w1147:dbl)
        n199 = call <vilib>:"Butterworth Filter PtByPt.vi"("initialize"="initialize", "order"="order", "filter type"="filter type", "low cutoff freq: fl"="low cutoff freq: fl", "high cutoff freq: fh"="high cutoff freq: fh", "sampling freq: fs"=w1171, "x"=w1164) -> ("Filtered x"=w1154:dbl)  [unwired: 2 in, 1 out]
        "Filtered Signal" <- w1154
        n200 = Exclusive Or(1:w1149, 2:w1150) -> (0:w1151:bool)
        n201 = Not(x=w1159) -> (.not. x?=w1160:bool)
        n202 = local read "Stop Button"() -> (w1143:bool)
        n203 = Or(x=w1160, y=w1151) -> (x .or. y?=w1139:bool)
        "Reset Fringe Counter" <- w1139
        n204 = call "Measure Fringe Displacement Simple.vi"("Photodiode Output"=w1154, "Fringe Counter Settings"="Fringe Counter Settings", "Reset"=w1139) -> ("Displacement"=w1157:dbl, "Input Signals"=→"Input Signals" →"Main Sig":dbl[][], "Stepped Signal"=→"Stepped Signal":dbl, "Output Signal"=→"Fringe Counter Output Signal":dbl[])  [unwired: 8 in, 1 out]
        "Relative Displacement" <- w1157
        n205 = case shown="True" w1159 {
          tunnel: w1147 -> [w1179 w1187]
          tunnel: [w1179 w1188] -> w1156
          tunnel: w1158 -> [_ w1183]
          tunnel: w1157 -> [_ w1185]
          tunnel: w1149 -> [w1178 w1184]
          tunnel: [w1178 w1184] -> w1152
          tunnel: w1139 -> [_ w1181]
          frame False {
          }
          frame True {
            n206 = Select(t=0.0, s=w1181, f=w1183) -> (s? t:f=w1182:dbl)
            n207 = Subtract(x=w1185, y=w1182) -> (x-y=w1186:dbl)
            n208 = case shown="False" w1184 {
              tunnel: [w1191 w1194] -> w1188
              tunnel: w1187 -> [w1189 w1193]
              tunnel: w1186 -> [w1190 w1192]
              frame False {
                n209 = Subtract(x=w1189, y=w1190) -> (x-y=w1191:dbl)
              }
              frame True {
                n210 = Add(x=w1193, y=w1192) -> (x+y=w1194:dbl)
              }
            }
          }
        }
        n211 = Or(x=w1142, y=w1143) -> (x .or. y?=w1144:bool)
        n212 = Reciprocal(x=w1171) -> (1/x=w1169:dbl)
        n213 = Multiply(x=1000.0 ("y"), y=w1169) -> (x*y=w1168:dbl)
        n214 = To Unsigned Long Integer(number=w1168) -> (unsigned 32bit integer=w1167:u32)
        n215 = Multiply(x=1000000.0, y=w1156) -> (x*y=→"Displacement" →"Total Displacement" →"Main Output":dbl)
        n216 = Wait Until Next ms Multiple(millisecond multiple=w1167) -> ()  [unwired: 1 out]
      }
      n217 = flat-sequence {
        tunnel: w880 -> [w906]
        tunnel: w879 -> [w905]
        tunnel: w878 -> [w904]
        tunnel: w877 -> [w901]
        tunnel: w874 -> [w899]
        tunnel: w873 -> [w898]
        frame #0 {
          n218 = call <userlib>:"stop motion.vi"("error in"=w905, "Axis in"=w906, "VISA Handle in"=w904) -> ("error out"=w903:errorcluster, "VISA Handle out"=w902:refnum<visa-resource-name>)  [unwired: 3 in, 2 out]
          n219 = call <userlib>:"Close.vi"("Error In"=w899, "LINX Resource"=w898) -> ("Error Out"=w900:errorcluster)  [unwired: 8 in, 1 out]
          n220 = call <vilib>:"Simple Error Handler.vi"("error in (no error)"=w900) -> ()  [unwired: 4 in, 5 out]
          n221 = call <userlib>:"stop motion.vi"("error in"=w903, "Axis in"=w901, "VISA Handle in"=w902) -> ("error out"=w913:errorcluster, "VISA Handle out"=w907:refnum<visa-resource-name>, "TimeoutFlag"=w910:bool)  [unwired: 3 in, 1 out]
          n222 = local write "Timeout"(w910) -> ()
          n223 = call "enter / leave remote mode.vi"("error in"=w913, "enter / disable remote mode (True)"=FALSE, "VISA handle in"=w907) -> ("error out"=w909:errorcluster, "VISA handle out"=w908:refnum<visa-resource-name>, "TimeoutFlag"=→"Timeout":bool)  [unwired: 6 in]
          n224 = call <userlib>:"close.vi"("VISA Handle in"=w908) -> ()  [unwired: 4 in, 1 out]
          n225 = call <vilib>:"General Error Handler.vi"("error in (no error)"=w909) -> ()  [unwired: 10 in, 5 out]
        }
        frame #1 {
          n226 = Stop() -> ()  [unwired: 1 in]
        }
      }
    }
  }
  n227 = case shown="True" w1 {
    frame False {
    }
    frame True {
      n228 = call <instrlib>:"Agilent E364X Series Output Single Channel DC Volts.vi"("VISA resource name"=refnum<visa-resource-name> "GPIB0::8::INSTR", "Output Enabled (False)"=TRUE, "Voltage Level (0.0 Volts)"=0.0, "Current Limit (0 Amps)"=0.0) -> ()  [unwired: 11 in, 1 out]
    }
  }
  n229 = case shown="True" w7 {
    tunnel: w22 -> [_ w1200]
    tunnel: w21 -> [_ w1199]
    frame False {
    }
    frame True {
      w1204 = 56 items=["No Error", "Argument Error", "Memory Full", "Out of Zone", "End of File", "File Already Open", "Generic File IO Error", "File Not Found", "File Permission Error", "Disk Full", "Duplicate Path", "Too Many Files Open", "Not Enabled", "Resource File Not Found", "Cannot Add Resource", "Resource Not Found", "Image Not Found", "Image Memory Error", "Pen Does Not Exist", "Config Bad Type", "Config Token Not Found", "Config Parse Error", "Config Memory Error", "Bad External Code Format", "Bad External Code Offset", "External Code Not Present", "Null Window", "Destroy Window Mixup", "Null Menu", "Print Aborted", "Bad Print Record", "Print Driver Error", "Windows Error During Print", "Memory Error During Print", "Print Dialog Error", "Generic Print Error", "Invalid Device Refnum", "Device Not Found", "Device Parameter Error", "Device Unit Error", "Can't Open Device", "Device Call Aborted", "Generic Error", "Cancelled By User", "Object ID Too Low", "Object ID Too High", "Object Not In Heap", "Unknown Heap", "Bad DefProc ID", "DefProc Not In Table", "Message Out Of Range", "Null Method", "Unknown Message", "Manager Call Not Supported", "Bad address", "Connection In progress", "Connection timed out", "Connection is already in progress", "Network attribute not supported", "Network error", "Address in use", "System out of memory", "Connection aborted", "Connection refused", "Connection is not connected", "Connection is already connected", "Connection closed", "Initialize error (interapplication manager)", "Bad occurrence", "Wait on unbound occurrence handler", "Occurrence queue overflow", "Bad path", "Semaphore not signaled", "Unrecognized type (interapplication manager)"] ("2nd Error to Convert")
      w1203 = 62 items=["No Error", "Argument Error", "Memory Full", "Out of Zone", "End of File", "File Already Open", "Generic File IO Error", "File Not Found", "File Permission Error", "Disk Full", "Duplicate Path", "Too Many Files Open", "Not Enabled", "Resource File Not Found", "Cannot Add Resource", "Resource Not Found", "Image Not Found", "Image Memory Error", "Pen Does Not Exist", "Config Bad Type", "Config Token Not Found", "Config Parse Error", "Config Memory Error", "Bad External Code Format", "Bad External Code Offset", "External Code Not Present", "Null Window", "Destroy Window Mixup", "Null Menu", "Print Aborted", "Bad Print Record", "Print Driver Error", "Windows Error During Print", "Memory Error During Print", "Print Dialog Error", "Generic Print Error", "Invalid Device Refnum", "Device Not Found", "Device Parameter Error", "Device Unit Error", "Can't Open Device", "Device Call Aborted", "Generic Error", "Cancelled By User", "Object ID Too Low", "Object ID Too High", "Object Not In Heap", "Unknown Heap", "Bad DefProc ID", "DefProc Not In Table", "Message Out Of Range", "Null Method", "Unknown Message", "Manager Call Not Supported", "Bad address", "Connection In progress", "Connection timed out", "Connection is already in progress", "Network attribute not supported", "Network error", "Address in use", "System out of memory", "Connection aborted", "Connection refused", "Connection is not connected", "Connection is already connected", "Connection closed", "Initialize error (interapplication manager)", "Bad occurrence", "Wait on unbound occurrence handler", "Occurrence queue overflow", "Bad path", "Semaphore not signaled", "Unrecognized type (interapplication manager)"] ("1st Error to Convert")
      n230 = TCP Close Connection(connection ID=w1199, error in (no error)=w1200) -> (error out=w1201:errorcluster)  [unwired: 1 in, 1 out]
      n231 = call <vilib>:"Error to Warning.vi"("1st Error to Convert"=w1203, "2nd Error to Convert"=w1204, "error in"=w1201) -> ("warning out"=w1202:errorcluster)  [unwired: 12 in]
      n232 = call <vilib>:"Simple Error Handler.vi"("error in (no error)"=w1202) -> ()  [unwired: 4 in, 5 out]
    }
  }
  n233 = case shown="True" w12 {
    tunnel: w14 -> [_ w1215]
    tunnel: w13 -> [_ w1214]
    frame False {
    }
    frame True {
      n234 = call "ag33xxx - Config Waveform.vi"("VISA session"=w1214, "Offset (0.00 V)"=0.0, "Frequency (1000 Hz)"=1000.0, "Amplitude (0.1 Vpp)"=1.0, "error in (no error)"=w1215) -> ("dup VISA session"=w1207:refnum<visa-resource-name>, "error out"=w1209:errorcluster)  [unwired: 9 in]
      n235 = call "ag33xxx - Error Query.vi"("error in (no error)"=w1209, "VISA session"=w1207) -> ("error out"=w1210:errorcluster, "dup VISA session"=w1211:refnum<visa-resource-name>)  [unwired: 6 in, 2 out]
      n236 = call "ag33xxx - Error Message.vi"("VISA session"=w1211, "error in (no error)"=w1210) -> ("dup VISA session"=w1206:refnum<visa-resource-name>, "error out"=w1208:errorcluster)  [unwired: 9 in, 3 out]
      n237 = call "ag33xxx - Close.vi"("error in (no error)"=w1208, "VISA session"=w1206) -> ()  [unwired: 9 in, 1 out]
    }
  }
